vi "Write Transfer Buffer.vi"(8 "error in (no error)":errorcluster, 9 "data":string, 10 "Transfer":refnum<class "Transfer.lvclass">, 11 "UDPlog Transceiver in":refnum<class "UDPlog Transceiver.lvclass">) -> (0 "error out":errorcluster, 3 "UDPlog Transceiver out":refnum<class "UDPlog Transceiver.lvclass">)   [LabVIEW 2023, in "UDPlog.lvlib" / "UDPlog Transceiver.lvclass"]
uses:
  UDPlog Transceiver.lvclass
  Users/Public/Documents/National Instruments/NI VeriStand 2023/Custom Devices/Data Sharing Framework/Linux_x64/DSF Core.lvlibp/Classes/Transfer/Transfer.lvclass
  Throw Size Mismatch Error.vi
  Users/Public/Documents/National Instruments/NI VeriStand 2023/Custom Devices/Data Sharing Framework/Linux_x64/DSF Core.lvlibp/Classes/Buffer/Write Buffer 1D U8.vi
  Users/Public/Documents/National Instruments/NI VeriStand 2023/Custom Devices/Data Sharing Framework/Linux_x64/DSF Core.lvlibp/Classes/Buffer/Buffer.lvclass
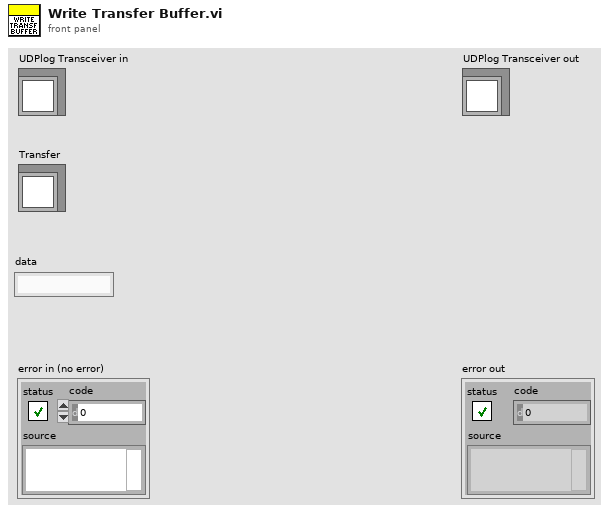
[diagram p1: front panel]
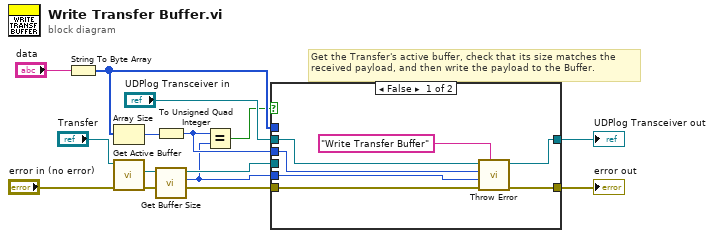
[diagram p0: block diagram]
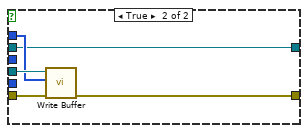
[diagram p2: hidden frame]
diagram:
  # "Get the Transfer's active buffer, check that its size matches the received payload, and then write the payload to the Buffer."
  n1 = String To Byte Array(string="data") -> (unsigned byte array=w8:u8[])
  n2 = Array Size(array=w8) -> (size(s)=w12:i32)
  n3 = call "Get Active Buffer.vi"("error in (no error)"="error in (no error)", "Transfer in"="Transfer") -> ("error out"=w6:errorcluster, "Buffer"=w10:refnum<class "Buffer.lvclass">)  [unwired: 7 in, 1 out]
  n4 = To Unsigned Quad Integer(1:w12) -> (0:w2:u64)
  n5 = call "Get Buffer Size.vi"("Buffer in"=w10) -> ("buffer size"=w1:u64, "Buffer out"=w5:refnum<class "Buffer.lvclass">)  [unwired: 9 in]
  n6 = Equal?(x=w2, y=w1) -> (x = y?=w7:bool)
  n7 = case shown="False" w7 {
    tunnel: "UDPlog Transceiver in" -> [w21 w22]
    tunnel: w8 -> [_ w24]
    tunnel: w6 -> [w16 w25]
    tunnel: w5 -> [_ w26]
    tunnel: [w15 w23] -> w4
    tunnel: [w20 w22] -> w3
    tunnel: w2 -> [w18 _]
    tunnel: w1 -> [w17 _]
    frame False {
      n8 = call-poly "Throw Error.vi"("source vi name"="Write Transfer Buffer", "error in (no error)"=w16, "actual size"=w17, "expected size"=w18, "UDP in"=w21) -> ("error out"=w15:errorcluster, "UDP out"=w20:refnum<class "UDPlog Transceiver.lvclass">)  [unwired: 5 in]
    }
    frame True {
      n9 = call-poly "Write Buffer.vi"("error in (no error)"=w25, "src array in"=w24, "Buffer in"=w26) -> ("error out"=w23:errorcluster)  [unwired: 5 in, 3 out]
    }
  }
  "error out" <- w4
  "UDPlog Transceiver out" <- w3
